vi "ConnectedStatus.vi"(8 "error in (no error)":errorcluster, 11 "NHRDCPower in":refnum<class "NHRDCPower.lvclass">) -> (0 "error out":errorcluster, 2 "Any Connections":bool, 3 "NHRDCPower out":refnum<class "NHRDCPower.lvclass">)   [LabVIEW 2018, in "AcPwrPlugins.lvlib" / "NHRDCPower.lvclass"]
doc: "This VI checks if the instrument has been connected and reports that value to any function calling it."
uses:
  NHRDCPower.lvclass
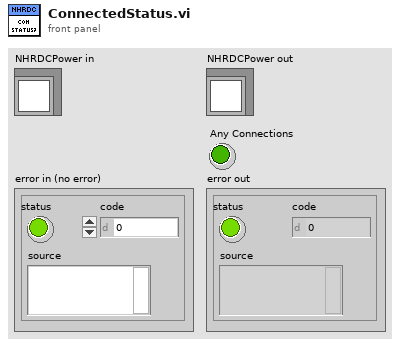
[diagram p1: front panel]
types:
  T1 = cluster{"Handle":string, "Name":string, "id query (Yes)":bool, "reset device (Yes)":bool, "Connected":bool, "Initial Battery Detect Voltage (0)":sgl, "SafetySettings":cluster{"SetWatchDog":bool, "Voltage (V)":sgl, "Current (A)":sgl, "Power (W)":sgl, "Voltage Delay (s)":sgl, "Current Delay (s)":sgl, "Power Delay (s)":sgl}, "Options String":string, "Aperture Time (s)":sgl, "operating state (Off)":i32, "OutputSettings":cluster{"Voltage (V)":sgl, "Current (A)":sgl, "Resistance (Ohms)":sgl, "Power (W)":sgl, "Enable Voltage":bool, "Enable Current":bool, "Enable Resistance":bool, "Enable Power":bool, "Delay After (s)":sgl, "Wait Value (V, A, W)":sgl, "Enable Wait":bool, "Wait on Value":i32}[], "SlewRate":cluster{"Set Voltage Rate V/S":dbl, "Set Current Rate A/S":dbl, "Set Resistance Rate R/S":dbl, "Set Power Rate W/S":dbl}}[]
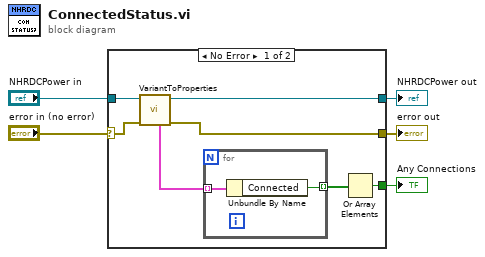
[diagram p0: block diagram]
diagram:
  n1 = case shown="No Error" "error in (no error)" {
    selector: "error in (no error)" -> [w9 w15]
    tunnel: "NHRDCPower in" -> [w10 w16]
    tunnel: [w7 w16] -> w3
    tunnel: [w8 w15] -> w2
    tunnel: [w11 _] -> w1
    frame No Error {
      n2 = call "VariantToProperties.vi"("error in (no error)"=w9, "NHRDCPower in"=w10) -> ("error out"=w8:errorcluster, "NHRDCPower out"=w7:refnum<class "NHRDCPower.lvclass">, "Modules"=w6:T1)  [unwired: 5 in, 2 out]
      n3 = for {
        tunnel: w6 -> [w14] mode=indexing
        tunnel: [w13] -> w12 mode=indexing
        n4 = Unbundle By Name(w14) -> ("Connected"=w13:bool)
      }
      n5 = Or Array Elements(Boolean array=w12) -> (logical OR=w11:bool)
    }
    frame Error {
    }
  }
  "error out" <- w2
  "NHRDCPower out" <- w3
  "Any Connections" <- w1
